vi "UserVars-Random Element of Expression.vi"(0 "Expr":string, 11 "error in (no error)":errorcluster) -> (4 "Random Element":dbl, 8 "Index":i32, 15 "error out":errorcluster)   [LabVIEW 2020]
uses:
  <vilib>/gmath/NI_Gmath.lvlib
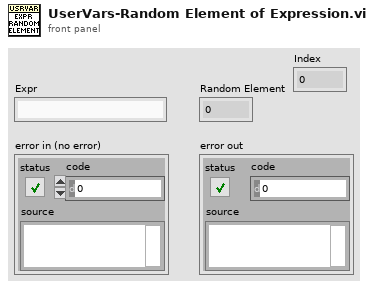
[diagram p1: front panel]
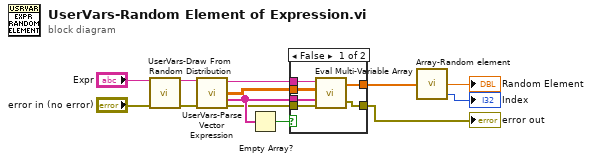
[diagram p0: block diagram]
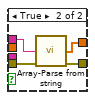
[diagram p2: hidden frame]
diagram:
  n1 = call "UserVars-Draw From Random Distribution.vi"("Expr in"="Expr", "error in (no error)"="error in (no error)") -> ("Expr out"=w3:string, "error out"=w2:errorcluster)  [unwired: 12 in]
  n2 = call "UserVars-Parse Vector Expression.vi"("Expression In"=w3, "error in (no error)"=w2) -> ("Expression Out"=w6:string, "values"=w7:dbl[][], "variables"=w12:string[], "error out"=w8:errorcluster)  [unwired: 10 in]
  n3 = Empty Array?(array=w12) -> (empty?=w13:bool)
  n4 = case shown="False" w13 {
    tunnel: w6 -> [w19 w22]
    tunnel: w7 -> [w18 _]
    tunnel: w12 -> [w17 _]
    tunnel: w8 -> [w16 w20]
    tunnel: [w15 w23] -> w9
    tunnel: [w14 w21] -> w10
    frame False {
      n5 = call <vilib>:"Eval Multi-Variable Array.vi"("error in (no error)"=w16, "Variables"=w17, "X Values"=w18, "formula"=w19) -> ("error out"=w15:errorcluster, "Y Values"=w14:dbl[])
    }
    frame True {
      n6 = call "Array-Parse from string.vi"("String"=w22, "error in (no error)"=w20) -> ("Array"=w21:dbl[], "error out"=w23:errorcluster)  [unwired: 12 in]
    }
  }
  "error out" <- w9
  n7 = call "Array-Random element.vi"("Array"=w10) -> ("Element"=→"Random Element":dbl, "Index"=→"Index":i32)  [unwired: 1 in]
